vi "1D Auto Correlation (CDB).vi"(10 "normalization":enum32{"none", "unbiased", "biased"}(ring), 11 "X":cdb[](array[numeric])) -> (0 "error":i32, 3 "Rxx":cdb[](array[numeric]))   [LabVIEW 2017, in "NI_AALPro.lvlib"]
doc: "Computes the autocorrelation of the input sequence <B>X</B>. Wire data to the <B>X</B> input to determine the polymorphic instance to use or manually select the instance."
uses:
  NI_AALPro.lvlib
  <resource>/lvanlys.dll
panel:
  # "1D AutoCorrelation (CDB)"
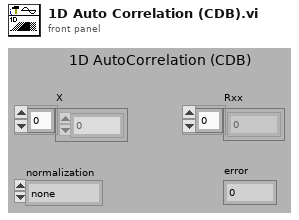
[diagram p1: front panel]
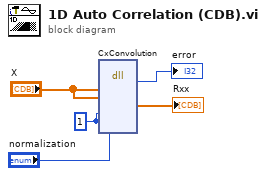
[diagram p0: block diagram]
diagram:
  w1 = 1 ("ConvOrCorr")
  n1 = dll-call lib="C:/Program Files (x86)/National Instruments/LabVIEW 2017/resource/lvanlys.*" fn="CxConvolution"("X"="X", "X"="X", "domain"=w1, "ConvOrCorr"=w1, "norm"="normalization") -> (→"error":i32, "Rxx"=→"Rxx":cdb[])  [unwired: 9 in, 2 out]
